vi "MAG_SW Final DVDD Voltage.vi"(7 "Waveform Array":waveform(dbl)[](array[waveform])) -> (8 "DVDD Voltage":dbl)   [LabVIEW 2010]
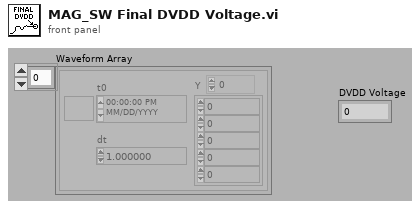
[diagram p1: front panel]
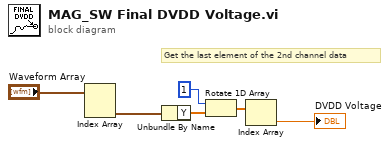
[diagram p0: block diagram]
diagram:
  # "Get the last element of the 2nd channel data"
  n1 = Index Array(array="Waveform Array") -> (element #2=w5:waveform(dbl))  [unwired: 2 in, 1 out]
  n2 = Unbundle By Name(w5) -> ("Y"=w4:dbl[])
  n3 = Rotate 1D Array(1:w4, 2:1 ("n")) -> (0:w2:dbl[])
  n4 = Index Array(array=w2) -> (element=→"DVDD Voltage":dbl)  [unwired: 1 in]
